vi "试验授权.vi"() -> ()   [LabVIEW 2016]
panel:
  out "布尔":bool
  in  "簇 3":T1
  out "簇":T1
  in  "R3加载时间/S  4":dbl=30.0
  in  "R2加载时间/S  4":dbl=30.0
  in  "R1加载时间/S  4":dbl=30.0
  in  "D6加载时间/S  4":dbl=30.0
  in  "D5加载时间/S  4":dbl=30.0
  in  "D4加载时间/S  4":dbl=30.0
  in  "D3加载时间/S 4":dbl=30.0
  in  "D2加载时间/S  4":dbl=30.0
  in  "D1加载时间/S 4":dbl=30.0
  in  "R3加载时间/S  3":dbl=30.0
  in  "R2加载时间/S  3":dbl=30.0
  in  "R1加载时间/S  3":dbl=30.0
  in  "D6加载时间/S  3":dbl=30.0
  in  "D5加载时间/S  3":dbl=30.0
  in  "D4加载时间/S  3":dbl=30.0
  in  "D3加载时间/S 3":dbl=30.0
  in  "D2加载时间/S  3":dbl=30.0
  in  "D1加载时间/S 3":dbl=30.0
  in  "R3加载时间/S  2":dbl=30.0
  in  "R2加载时间/S  2":dbl=30.0
  in  "R1加载时间/S  2":dbl=30.0
  in  "D6加载时间/S  2":dbl=30.0
  in  "D5加载时间/S  2":dbl=30.0
  in  "D4加载时间/S  2":dbl=30.0
  in  "D3加载时间/S 2":dbl=30.0
  in  "D2加载时间/S  2":dbl=30.0
  in  "D1加载时间/S 2":dbl=30.0
  in  "SG18-3百分比":dbl min=0.0 max=100.0 step=1.0
  in  "SG16-3百分比":dbl min=0.0 max=100.0 step=1.0
  in  "SG14百分比":dbl min=0.0 max=100.0 step=1.0
  in  "R3加载时间/S":dbl=30.0
  in  "R2加载时间/S":dbl=30.0
  in  "R1加载时间/S":dbl=30.0
  in  "D6加载时间/S":dbl=30.0
  in  "D5加载时间/S":dbl=30.0
  in  "D4加载时间/S":dbl=30.0
  in  "D3加载时间/S":dbl=30.0
  in  "D2加载时间/S":dbl=30.0
  in  "D1加载时间/S":dbl=30.0
  in  "R3":dbl min=0.0 max=100.0 step=1.0
  in  "R2":dbl min=0.0 max=100.0 step=1.0
  in  "R1":dbl min=0.0 max=100.0 step=1.0
  in  "D6":dbl min=0.0 max=100.0 step=1.0
  in  "D5":dbl min=0.0 max=100.0 step=1.0
  in  "D4":dbl min=0.0 max=100.0 step=1.0
  in  "D3":dbl=30.0 min=0.0 max=100.0 step=1.0
  in  "D2":dbl=50.0 min=0.0 max=100.0 step=1.0
  in  "D1":dbl=50.0 min=0.0 max=100.0 step=1.0
  in  "确定按钮":bool
  # "SG21时间"
  # "SG14时间"
  # "SG16时间"
  # "SG18时间"
  # "百分比"
  # "百分比"
  # "百分比"
  # "百分比"
  # "百分比"
  # "百分比"
  # "百分比"
  # "百分比"
  # "百分比"
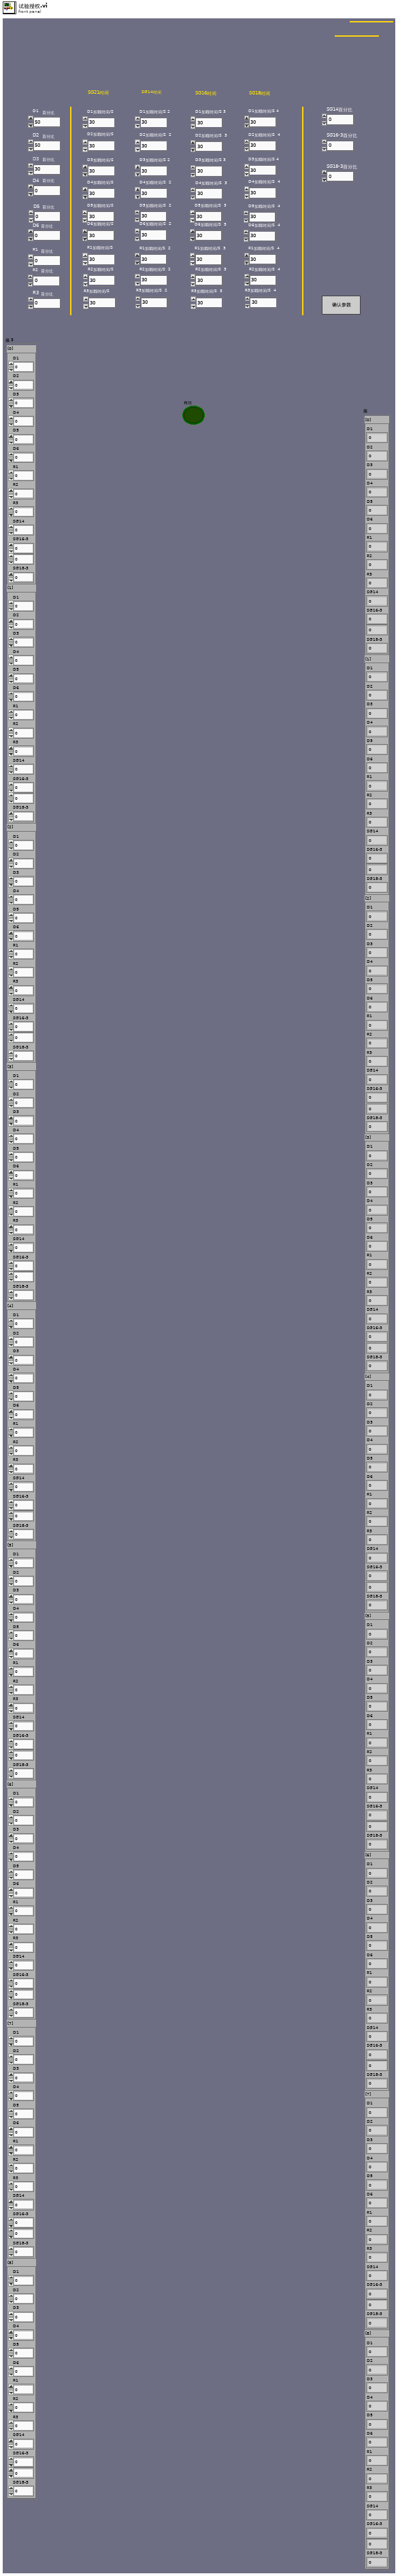
[diagram p1: front panel]
types:
  T1 = cluster{"[0]":cluster{"D1":dbl, "D2":dbl, "D3":dbl, "D4":dbl, "D5":dbl, "D6":dbl, "R1":dbl, "R2":dbl, "R3":dbl, "SG14":dbl, "SG16-3":dbl, dbl, "SG18-3 ":dbl}, "[1]":cluster{"D1":dbl, "D2":dbl, "D3":dbl, "D4":dbl, "D5":dbl, "D6":dbl, "R1":dbl, "R2":dbl, "R3":dbl, "SG14":dbl, "SG16-3":dbl, dbl, "SG18-3 ":dbl}, "[2]":cluster{"D1":dbl, "D2":dbl, "D3":dbl, "D4":dbl, "D5":dbl, "D6":dbl, "R1":dbl, "R2":dbl, "R3":dbl, "SG14":dbl, "SG16-3":dbl, dbl, "SG18-3 ":dbl}, "[3]":cluster{"D1":dbl, "D2":dbl, "D3":dbl, "D4":dbl, "D5":dbl, "D6":dbl, "R1":dbl, "R2":dbl, "R3":dbl, "SG14":dbl, "SG16-3":dbl, dbl, "SG18-3 ":dbl}, "[4]":cluster{"D1":dbl, "D2":dbl, "D3":dbl, "D4":dbl, "D5":dbl, "D6":dbl, "R1":dbl, "R2":dbl, "R3":dbl, "SG14":dbl, "SG16-3":dbl, dbl, "SG18-3 ":dbl}, "[5]":cluster{"D1":dbl, "D2":dbl, "D3":dbl, "D4":dbl, "D5":dbl, "D6":dbl, "R1":dbl, "R2":dbl, "R3":dbl, "SG14":dbl, "SG16-3":dbl, dbl, "SG18-3 ":dbl}, "[6]":cluster{"D1":dbl, "D2":dbl, "D3":dbl, "D4":dbl, "D5":dbl, "D6":dbl, "R1":dbl, "R2":dbl, "R3":dbl, "SG14":dbl, "SG16-3":dbl, dbl, "SG18-3 ":dbl}, "[7]":cluster{"D1":dbl, "D2":dbl, "D3":dbl, "D4":dbl, "D5":dbl, "D6":dbl, "R1":dbl, "R2":dbl, "R3":dbl, "SG14":dbl, "SG16-3":dbl, dbl, "SG18-3 ":dbl}, "[8]":cluster{"D1":dbl, "D2":dbl, "D3":dbl, "D4":dbl, "D5":dbl, "D6":dbl, "R1":dbl, "R2":dbl, "R3":dbl, "SG14":dbl, "SG16-3":dbl, dbl, "SG18-3 ":dbl}}
  T2 = cluster{"[0]":cluster{"D1":dbl, "D2":dbl, "D3":dbl, "D4":dbl, "D5":dbl, "D6":dbl, "R1":dbl, "R2":dbl, "R3":dbl, "SG14":dbl, "SG16-3":dbl, dbl, "SG18-3 ":dbl}, "[1]":cluster{"D1":dbl, "D2":dbl, "D3":dbl, "D4":dbl, "D5":dbl, "D6":dbl, "R1":dbl, "R2":dbl, "R3":dbl, "SG14":dbl, "SG16-3":dbl, dbl, "SG18-3 ":dbl}, "[2]":cluster{"D1":dbl, "D2":dbl, "D3":dbl, "D4":dbl, "D5":dbl, "D6":dbl, "R1":dbl, "R2":dbl, "R3":dbl, "SG14":dbl, "SG16-3":dbl, dbl, "SG18-3 ":dbl}, "[3]":cluster{"D1":dbl, "D2":dbl, "D3":dbl, "D4":dbl, "D5":dbl, "D6":dbl, "R1":dbl, "R2":dbl, "R3":dbl, "SG14":dbl, "SG16-3":dbl, dbl, "SG18-3 ":dbl}, "[4]":cluster{"D1":dbl, "D2":dbl, "D3":dbl, "D4":dbl, "D5":dbl, "D6":dbl, "R1":dbl, "R2":dbl, "R3":dbl, "SG14":dbl, "SG16-3":dbl, dbl, "SG18-3 ":dbl}, "[5]":cluster{"D1":dbl, "D2":dbl, "D3":dbl, "D4":dbl, "D5":dbl, "D6":dbl, "R1":dbl, "R2":dbl, "R3":dbl, "SG14":dbl, "SG16-3":dbl, dbl, "SG18-3 ":dbl}, "[6]":cluster{"D1":dbl, "D2":dbl, "D3":dbl, "D4":dbl, "D5":dbl, "D6":dbl, "R1":dbl, "R2":dbl, "R3":dbl, "SG14":dbl, "SG16-3":dbl, dbl, "SG18-3 ":dbl}, "[7]":cluster{"D1":dbl, "D2":dbl, "D3":dbl, "D4":dbl, "D5":dbl, "D6":dbl, "R1":dbl, "R2":dbl, "R3":dbl, "SG14":dbl, "SG16-3":dbl, dbl, "SG18-3 ":dbl}, "[8]":cluster{"D1":dbl, "D2":dbl, "D3":dbl, "D4":dbl, "D5":dbl, "D6":dbl, "R1":dbl, "R2":dbl, "R3":dbl, "SG14":dbl, "SG16-3":dbl, dbl, "SG18-3 ":dbl}}[]
  T3 = cluster{"D1":dbl, "D2":dbl, "D3":dbl, "D4":dbl, "D5":dbl, "D6":dbl, "R1":dbl, "R2":dbl, "R3":dbl, "SG14":dbl, "SG16-3":dbl, dbl, "SG18-3 ":dbl}
  T4 = cluster{"D1":dbl, "D2":dbl, "D3":dbl, "D4":dbl, "D5":dbl, "D6":dbl, "R1":dbl, "R2":dbl, "R3":dbl, "SG14":dbl, "SG16-3":dbl, dbl, "SG18-3 ":dbl}[]
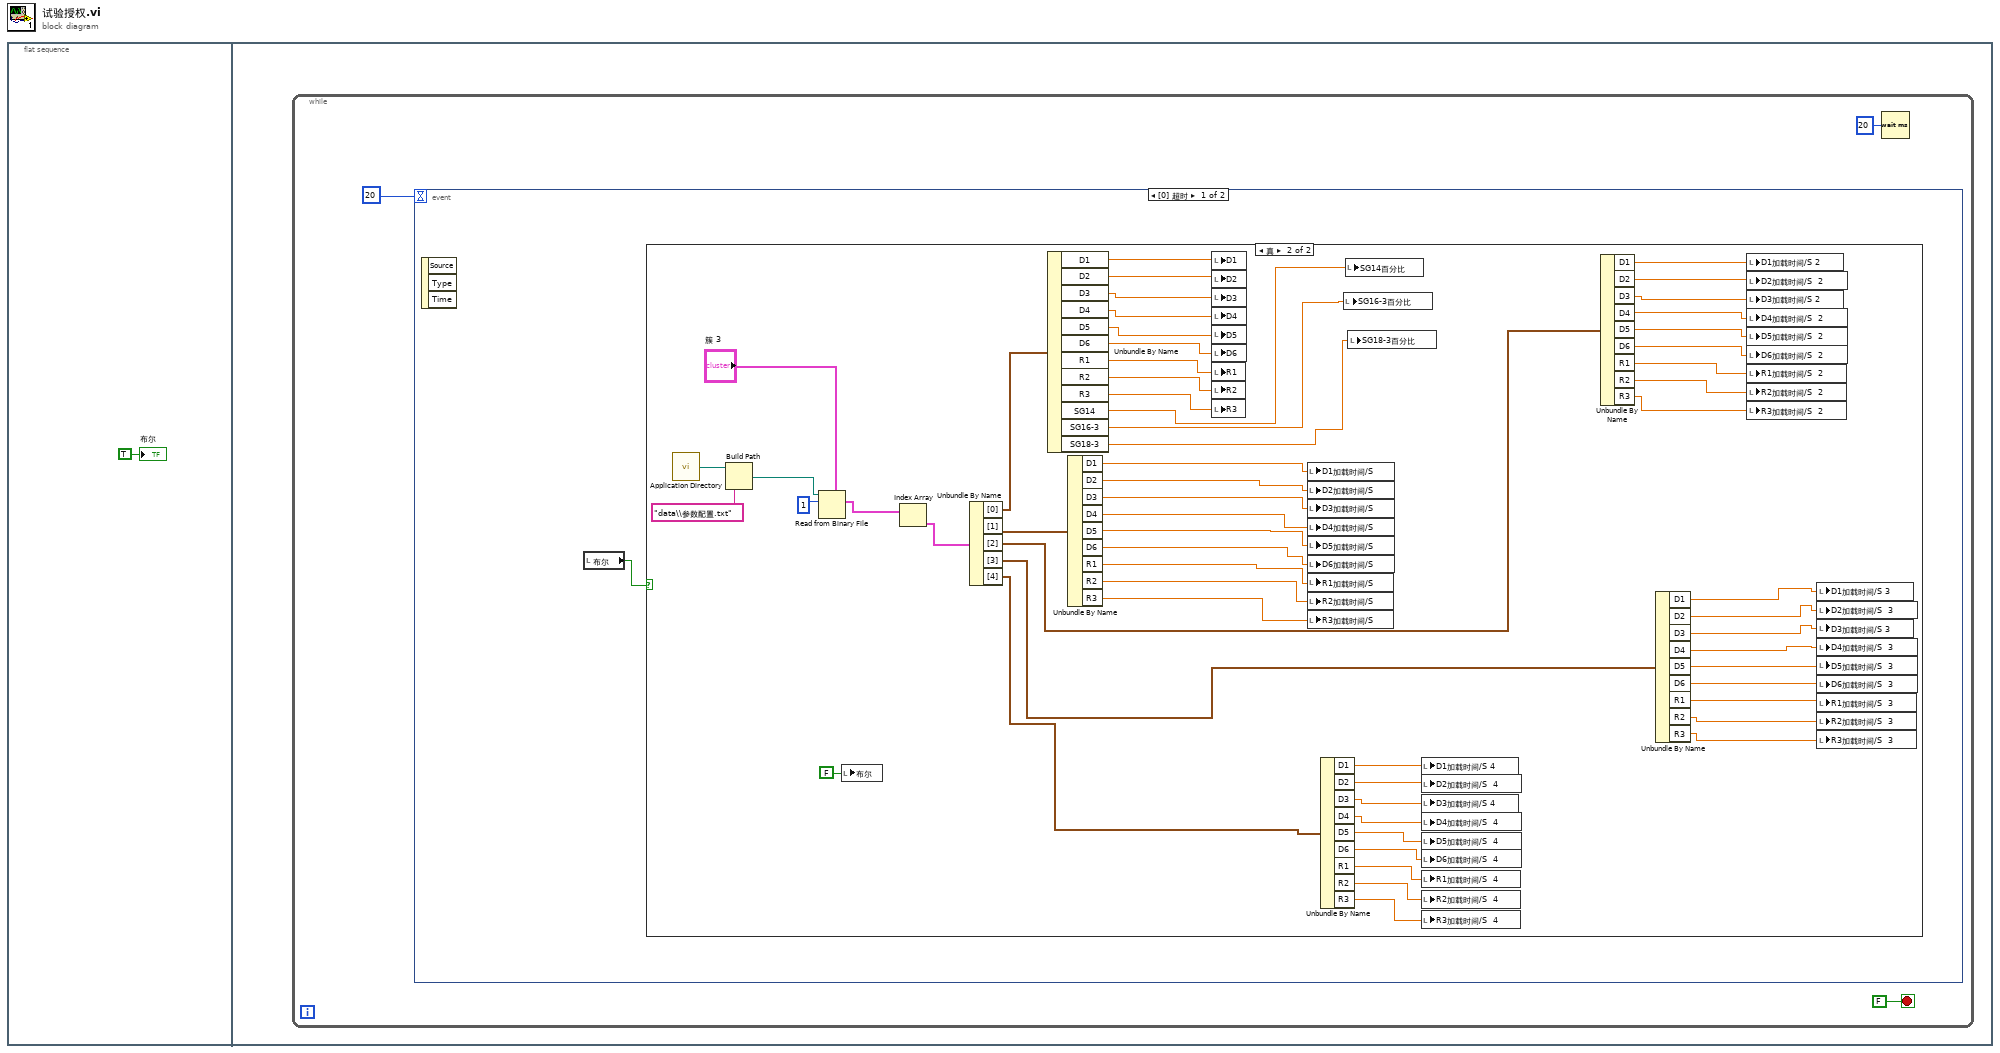
[diagram p0: block diagram]
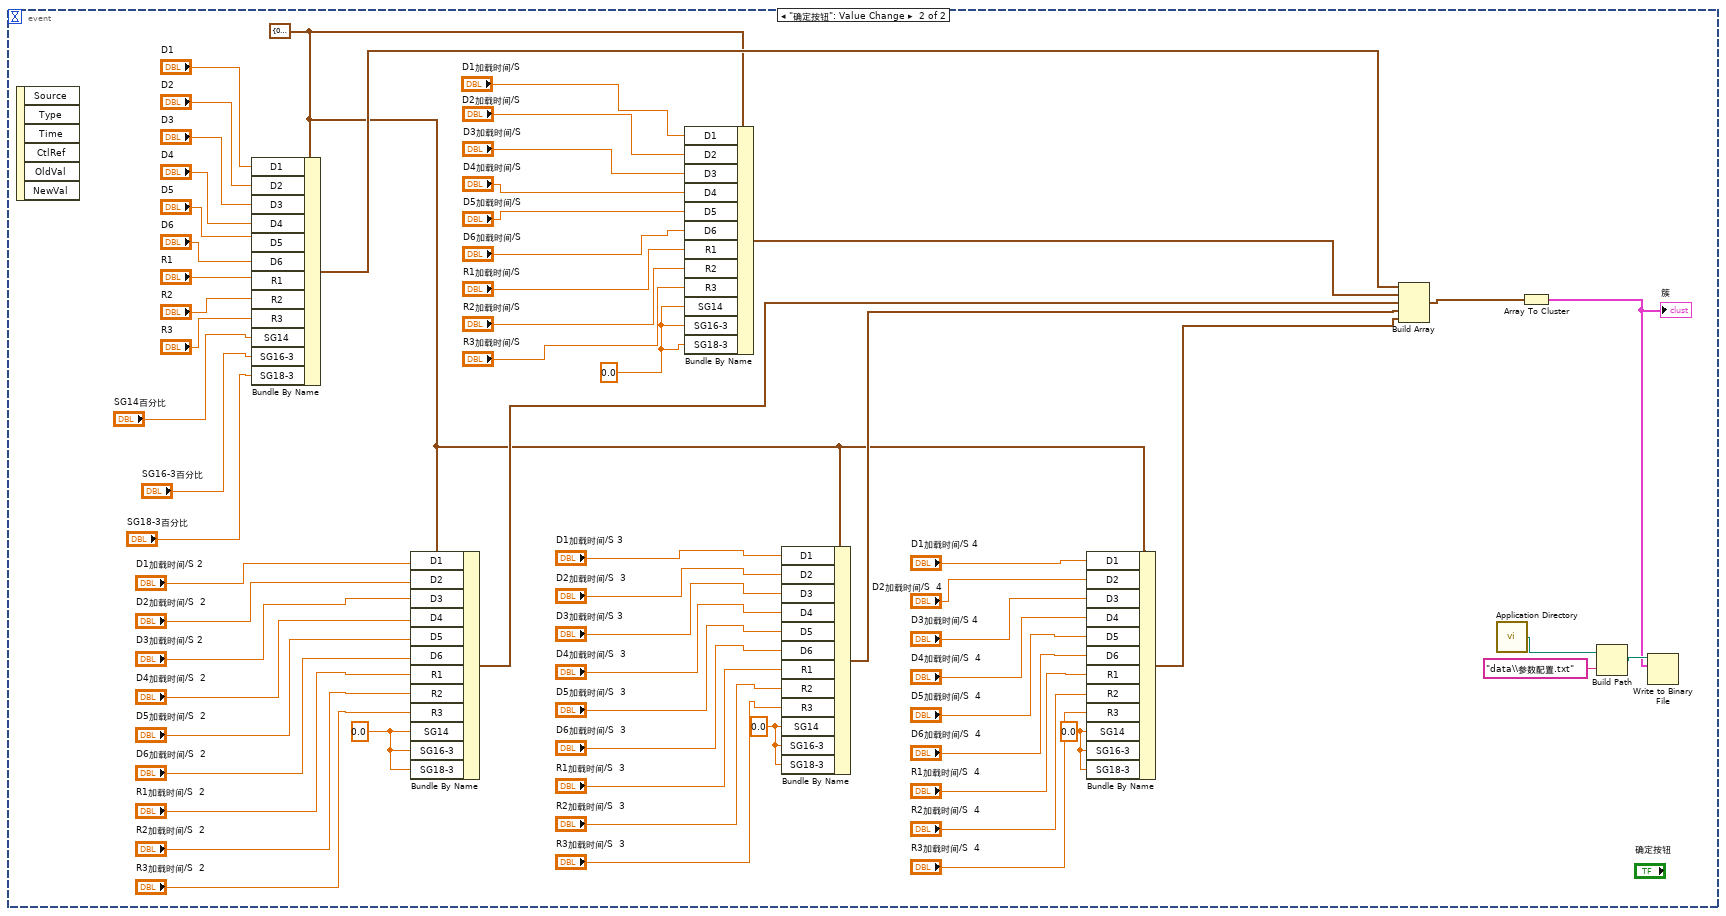
[diagram p3: hidden frame]
diagram:
  n1 = flat-sequence {
    frame #0 {
      "布尔" <- TRUE ("布尔")
    }
    frame #1 {
      n2 = while {
        stop <- FALSE stop-if-true
        n3 = event shown="[0] 超时" {
          selector: _ -> [_ _]
          dyn-events: _ -> [_ _]
          timeout: 20 -> [_ _]
          event Timeout {
            n4 = event-data() -> ()  [unwired: 1 in, 3 out]
            n5 = local read "布尔"() -> (w5:bool)
            n6 = case shown="真" w5 {
              frame False {
              }
              frame True {
                n7 = call <vilib>:"Application Directory.vi"() -> ("Application Directory"=w65:path)
                n8 = Build Path(base path=w65, name or relative path="data\\参数配置.txt" ("名称或相对路径")) -> (appended path=w63:path)
                n9 = Read from Binary File(5:"簇 3", 10:1 ("总数(1)"), 11:w63) -> (2:w61:T2)  [unwired: 3 in, 3 out]
                n10 = local write "布尔"(FALSE ("布尔")) -> ()
                n11 = Index Array(array=w61) -> (element=w60:T1)  [unwired: 1 in]
                n12 = Unbundle By Name(w60) -> ("[0]"=w59:T3, "[1]"=w46:T3, "[2]"=w36:T3, "[3]"=w35:T3, "[4]"=w16:T3)
                n13 = Unbundle By Name(w59) -> ("D1"=w58:dbl, "D2"=w57:dbl, "D3"=w56:dbl, "D4"=w55:dbl, "D5"=w54:dbl, "D6"=w53:dbl, "R1"=w52:dbl, "R2"=w51:dbl, "R3"=w50:dbl, "SG14"=w49:dbl, "SG16-3"=w48:dbl, "SG18-3"=w47:dbl)
                n14 = Unbundle By Name(w46) -> ("D1"=w45:dbl, "D2"=w44:dbl, "D3"=w43:dbl, "D4"=w42:dbl, "D5"=w41:dbl, "D6"=w40:dbl, "R1"=w39:dbl, "R2"=w38:dbl, "R3"=w37:dbl)
                n15 = local write "D1"(w58) -> ()
                n16 = local write "D2"(w57) -> ()
                n17 = local write "D3"(w56) -> ()
                n18 = local write "D4"(w55) -> ()
                n19 = local write "D5"(w54) -> ()
                n20 = local write "D6"(w53) -> ()
                n21 = local write "R1"(w52) -> ()
                n22 = local write "R2"(w51) -> ()
                n23 = local write "R3"(w50) -> ()
                n24 = local write "D1加载时间/S"(w45) -> ()
                n25 = local write "D2加载时间/S"(w44) -> ()
                n26 = local write "D3加载时间/S"(w43) -> ()
                n27 = local write "D4加载时间/S"(w42) -> ()
                n28 = local write "D5加载时间/S"(w41) -> ()
                n29 = local write "D6加载时间/S"(w40) -> ()
                n30 = local write "R1加载时间/S"(w39) -> ()
                n31 = local write "R2加载时间/S"(w38) -> ()
                n32 = local write "R3加载时间/S"(w37) -> ()
                n33 = Unbundle By Name(w16) -> ("D1"=w15:dbl, "D2"=w14:dbl, "D3"=w13:dbl, "D4"=w12:dbl, "D5"=w11:dbl, "D6"=w10:dbl, "R1"=w9:dbl, "R2"=w8:dbl, "R3"=w7:dbl)
                n34 = local write "SG16-3百分比"(w48) -> ()
                n35 = local write "SG14百分比"(w49) -> ()
                n36 = local write "SG18-3百分比"(w47) -> ()
                n37 = local write "D1加载时间/S 4"(w15) -> ()
                n38 = local write "D2加载时间/S  4"(w14) -> ()
                n39 = local write "D3加载时间/S 4"(w13) -> ()
                n40 = local write "D4加载时间/S  4"(w12) -> ()
                n41 = local write "D5加载时间/S  4"(w11) -> ()
                n42 = local write "D6加载时间/S  4"(w10) -> ()
                n43 = local write "R1加载时间/S  4"(w9) -> ()
                n44 = local write "R2加载时间/S  4"(w8) -> ()
                n45 = local write "R3加载时间/S  4"(w7) -> ()
                n46 = Unbundle By Name(w36) -> ("D1"=w34:dbl, "D2"=w33:dbl, "D3"=w32:dbl, "D4"=w31:dbl, "D5"=w30:dbl, "D6"=w29:dbl, "R1"=w28:dbl, "R2"=w27:dbl, "R3"=w26:dbl)
                n47 = Unbundle By Name(w35) -> ("D1"=w25:dbl, "D2"=w24:dbl, "D3"=w23:dbl, "D4"=w22:dbl, "D5"=w21:dbl, "D6"=w20:dbl, "R1"=w19:dbl, "R2"=w18:dbl, "R3"=w17:dbl)
                n48 = local write "D1加载时间/S 2"(w34) -> ()
                n49 = local write "D2加载时间/S  2"(w33) -> ()
                n50 = local write "D3加载时间/S 2"(w32) -> ()
                n51 = local write "D4加载时间/S  2"(w31) -> ()
                n52 = local write "D5加载时间/S  2"(w30) -> ()
                n53 = local write "D6加载时间/S  2"(w29) -> ()
                n54 = local write "R1加载时间/S  2"(w28) -> ()
                n55 = local write "R2加载时间/S  2"(w27) -> ()
                n56 = local write "R3加载时间/S  2"(w26) -> ()
                n57 = local write "D1加载时间/S 3"(w25) -> ()
                n58 = local write "D2加载时间/S  3"(w24) -> ()
                n59 = local write "D3加载时间/S 3"(w23) -> ()
                n60 = local write "D4加载时间/S  3"(w22) -> ()
                n61 = local write "D5加载时间/S  3"(w21) -> ()
                n62 = local write "D6加载时间/S  3"(w20) -> ()
                n63 = local write "R1加载时间/S  3"(w19) -> ()
                n64 = local write "R2加载时间/S  3"(w18) -> ()
                n65 = local write "R3加载时间/S  3"(w17) -> ()
              }
            }
          }
          event "确定按钮": Value Change {
            w69 = 0.0 ("SG14")
            w81 = 0.0 ("SG14")
            w92 = 0.0 ("SG14")
            w102 = 0.0 ("SG14")
            w79 = T3 {"D1"=0.0, "D2"=0.0, "D3"=0.0, "D4"=0.0, "D5"=0.0, "D6"=0.0, "R1"=0.0, "R2"=0.0, "R3"=0.0, "SG14"=0.0, "SG16-3"=0.0, 0.0, "SG18-3 "=0.0}
            n66 = event-data() -> ()  [unwired: 1 in, 6 out]
            n67 = Bundle By Name(cluster=w79, "D1"="D1", "D2"="D2", "D3"="D3", "D4"="D4", "D5"="D5", "D6"="D6", "R1"="R1", "R2"="R2", "R3"="R3", "SG14"="SG14百分比", "SG16-3"="SG16-3百分比", "SG18-3"="SG18-3百分比") -> (w111:T3)
            n68 = Bundle By Name(cluster=w79, "D1"="D1加载时间/S 2", "D2"="D2加载时间/S  2", "D3"="D3加载时间/S 2", "D4"="D4加载时间/S  2", "D5"="D5加载时间/S  2", "D6"="D6加载时间/S  2", "R1"="R1加载时间/S  2", "R2"="R2加载时间/S  2", "R3"="R3加载时间/S  2", "SG14"=w92, "SG16-3"=w92, "SG18-3"=w92) -> (w91:T3)
            n69 = Bundle By Name(cluster=w79, "D1"="D1加载时间/S", "D2"="D2加载时间/S", "D3"="D3加载时间/S", "D4"="D4加载时间/S", "D5"="D5加载时间/S", "D6"="D6加载时间/S", "R1"="R1加载时间/S", "R2"="R2加载时间/S", "R3"="R3加载时间/S", "SG14"=w102, "SG16-3"=w102, "SG18-3"=w102) -> (w110:T3)
            n70 = Bundle By Name(cluster=w79, "D1"="D1加载时间/S 3", "D2"="D2加载时间/S  3", "D3"="D3加载时间/S 3", "D4"="D4加载时间/S  3", "D5"="D5加载时间/S  3", "D6"="D6加载时间/S  3", "R1"="R1加载时间/S  3", "R2"="R2加载时间/S  3", "R3"="R3加载时间/S  3", "SG14"=w81, "SG16-3"=w81, "SG18-3"=w81) -> (w80:T3)
            n71 = Bundle By Name(cluster=w79, "D1"="D1加载时间/S 4", "D2"="D2加载时间/S  4", "D3"="D3加载时间/S 4", "D4"="D4加载时间/S  4", "D5"="D5加载时间/S  4", "D6"="D6加载时间/S  4", "R1"="R1加载时间/S  4", "R2"="R2加载时间/S  4", "R3"="R3加载时间/S  4", "SG14"=w69, "SG16-3"=w69, "SG18-3"=w69) -> (w68:T3)
            n72 = Build Array(w111, w110, w91, w80, w68) -> (w106:T4)
            n73 = call <vilib>:"Application Directory.vi"() -> ("Application Directory"=w109:path)
            n74 = Array To Cluster(array=w106) -> (cluster=w67:T1)
            "簇" <- w67
            n75 = Build Path(base path=w109, name or relative path="data\\参数配置.txt" ("名称或相对路径")) -> (appended path=w107:path)
            n76 = Write to Binary File(file (use dialog)=w107, data=w67) -> ()  [unwired: 4 in, 3 out]
          }
        }
        n77 = Wait (ms)(milliseconds to wait=u32 20 ("等待时间（毫秒）")) -> ()  [unwired: 1 out]
      }
    }
  }
